vi "AI_all.vi"() -> ()   [LabVIEW 2019]
panel:
  out "Waveform Chart":T1(graph)
  out "AI float":sgl[](array[numeric]) format="%.2f"
  in  "BaudRate":u32=115200
  out "return":i16
  in  "DCON_AI_Module":T2={"ComPort"=1, "Address"=1, "Slot"=1, "CheckSum"=0, "TimeOut"=1000}
  in  "stop":bool
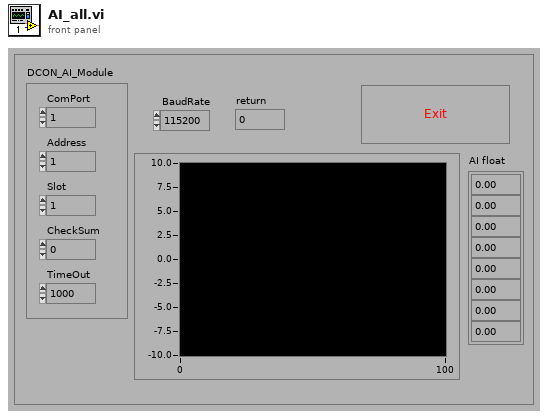
[diagram p1: front panel]
types:
  T1 = cluster{"Float_AI":sgl, "Float_AI":sgl, "Float_AI":sgl, "Float_AI":sgl, "Float_AI":sgl, "Float_AI":sgl, "Float_AI":sgl, "Float_AI":sgl}
  T2 = cluster{"ComPort":u8, "Address":i16, "Slot":i16, "CheckSum":i16, "TimeOut":i16}
  T3 = cluster{"AI float[0]":sgl, "AI float[1]":sgl, "AI float[2]":sgl, "AI float[3]":sgl, "AI float[4]":sgl, "AI float[5]":sgl, "AI float[6]":sgl, "AI float[7]":sgl}
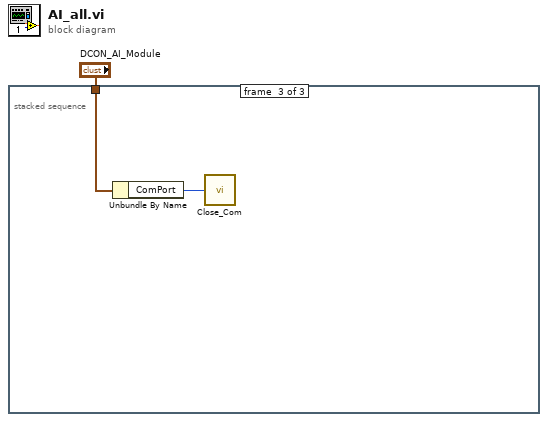
[diagram p0: block diagram]
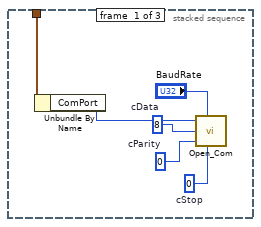
[diagram p2: hidden frame]
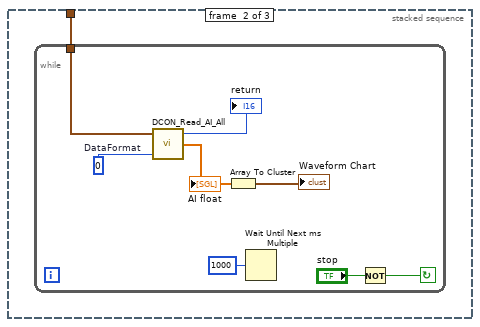
[diagram p3: hidden frame]
diagram:
  n1 = stacked-sequence {
    tunnel: "DCON_AI_Module" -> [w4 w8 w18]
    frame #0 {
      w5 = u8 0  # cStop
      w6 = u8 0  # cParity
      w7 = u8 8  # cData
      n2 = Unbundle By Name(w4) -> ("ComPort"=w3:u8)
      n3 = call "Open_Com.VI"("port number"=w3, "baudrate (115200)"="BaudRate", "data bit (8)"=w7, "parity (0: none)"=w6, "stop bit (0: 1 stop bit)"=w5) -> ()  [unwired: 1 out]
    }
    frame #1 {
      n4 = while {
        tunnel: w8 -> [w13]
        stop <- w16 continue-if-true
        w12 = i16 0  # DataFormat
        n5 = call "DCON_Read_AI_All.vi"("DataFormat (0)"=w12, "DCON_Module"=w13) -> ("AI float"=w10:sgl[], "return"=→"return":i16)  [unwired: 1 in, 1 out]
        "AI float" <- w10
        n6 = Array To Cluster(array=w10) -> (cluster=→"Waveform Chart":T3)
        n7 = Wait Until Next ms Multiple(millisecond multiple=u32 1000) -> ()  [unwired: 1 out]
        n8 = Not(x="stop") -> (.not. x?=w16:bool)
      }
    }
    frame #2 {
      n9 = Unbundle By Name(w18) -> ("ComPort"=w17:u8)
      n10 = call "Close_Com.vi"("port number"=w17) -> ()  [unwired: 1 out]
    }
  }
